vi "Light Info.vi"(8 "error in (no error)":errorcluster, 10 "Light Name":string, 11 "FlexWorktable in":refnum<class "FlexWorktable.lvclass">) -> (0 "error out":errorcluster, 1 "hardware_address":string, 2 "control":string, 3 "FlexWorktable out":refnum<class "FlexWorktable.lvclass">)   [LabVIEW 2017, in "FlexWorktable.lvclass"]
uses:
  FlexWorktable.lvclass
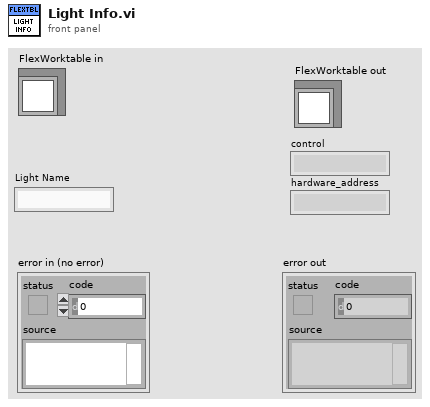
[diagram p1: front panel]
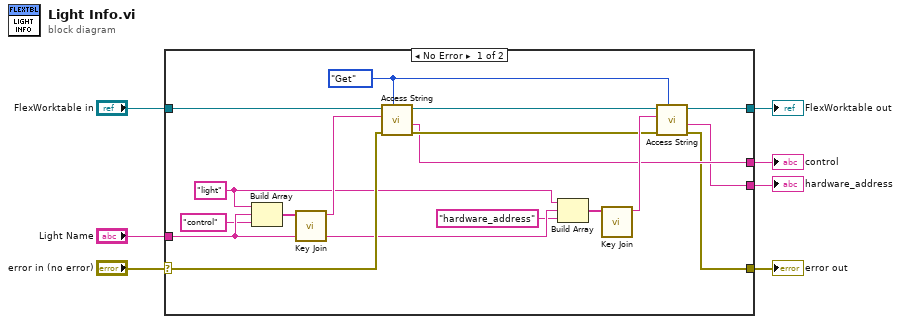
[diagram p0: block diagram]
diagram:
  n1 = case shown="No Error" "error in (no error)" {
    selector: "error in (no error)" -> [w19 w26]
    tunnel: [w9 w26] -> w6
    tunnel: [w8 w25] -> w4
    tunnel: "FlexWorktable in" -> [w24 w25]
    tunnel: "Light Name" -> [w17 _]
    tunnel: [w11 _] -> w2
    tunnel: [w10 _] -> w1
    frame No Error {
      w16 = "light" ("element")
      w22 = enum16{"Get", "Set"}."Get" ("Get/Set")
      n2 = Build Array(w16, w17, "control" ("element")) -> (w21:string[])
      n3 = call "Key Join.vi"("Key Elements"=w21) -> ("Key"=w20:string)  [unwired: 10 in]
      n4 = call-dynamic "Access String.vi"("Get/Set"=w22, "error in (no error)"=w19, "Key"=w20, "FlexWorktable in"=w24) -> ("error out"=w12:errorcluster, "Value out"=w11:string, "FlexWorktable out"=w23:refnum<class "FlexWorktable.lvclass">)  [unwired: 5 in]
      n5 = Build Array(w16, w17, "hardware_address" ("element")) -> (w18:string[])
      n6 = call "Key Join.vi"("Key Elements"=w18) -> ("Key"=w13:string)  [unwired: 10 in]
      n7 = call-dynamic "Access String.vi"("Get/Set"=w22, "error in (no error)"=w12, "Key"=w13, "FlexWorktable in"=w23) -> ("error out"=w9:errorcluster, "Value out"=w10:string, "FlexWorktable out"=w8:refnum<class "FlexWorktable.lvclass">)  [unwired: 5 in]
    }
    frame Error {
    }
  }
  "error out" <- w6
  "FlexWorktable out" <- w4
  "control" <- w2
  "hardware_address" <- w1
